vi "1 Tap 36-Bit RGB.vi"() -> ()   [LabVIEW 2012]
uses:
  <vilib>/rvi/eio/common/nirviEmuTemplateMethod_errors.vi
  <vilib>/eio/EIONode/EIONode.xnode
panel:
  out "PixelData":u64
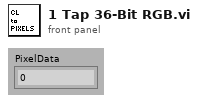
[diagram p1: front panel]
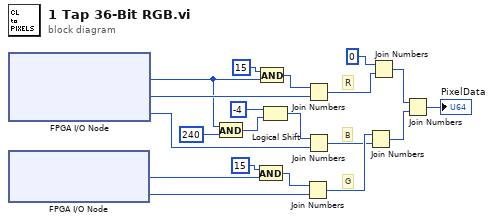
[diagram p0: block diagram]
diagram:
  # "B"
  # "R"
  # "G"
  n1 = xnode "FPGA I/O Node"() -> ("IO Module\\CL Port B"=w5:u8, "IO Module\\CL Port A"=w15:u8, "IO Module\\CL Port C"=w9:u8)  [unwired: 3 in, 3 out]
  n2 = xnode "FPGA I/O Node"() -> ("IO Module\\CL Port F"=w12:u8, "IO Module\\CL Port E"=w11:u8)  [unwired: 2 in, 2 out]
  n3 = And(x=w5, y=u8 240 ("hi")) -> (x .and. y?=w18:u8)
  n4 = And(x=u8 15 ("hi"), y=w12) -> (x .and. y?=w14:u8)
  n5 = And(x=u8 15 ("hi"), y=w5) -> (x .and. y?=w19:u8)
  n6 = Logical Shift(y=i8 -4, x=w18) -> (x << y=w16:u8)
  n7 = Join Numbers(hi=w14, lo=w11) -> ((hi.lo)=w8:u16)
  n8 = Join Numbers(hi=w19, lo=w15) -> ((hi.lo)=w10:u16)
  n9 = Join Numbers(hi=w16, lo=w9) -> ((hi.lo)=w7:u16)
  n10 = Join Numbers(hi=w8, lo=w7) -> ((hi.lo)=w1:u32)
  n11 = Join Numbers(hi=u16 0, lo=w10) -> ((hi.lo)=w3:u32)
  n12 = Join Numbers(hi=w3, lo=w1) -> ((hi.lo)=→"PixelData":u64)
